vi "tlc_timer_main.vi"(7 "Command (Check Timer)":T1=enum."Check Timer", 8 "error in (no error)":errorcluster, 11 "Target Time (s)":dbl) -> (0 "error out":errorcluster, 3 "Elapsed":bool)   [LabVIEW 2009]
doc: "This VI is the Main VI for the Timer module. The Timer module is responsible for checking whether the Target Time has Elapsed.\n\nSee Block Diagram for more detailed information."
uses:
  tlc_timer_Command_enum.ctl
panel:
  # "Inputs"
  # "Outputs"
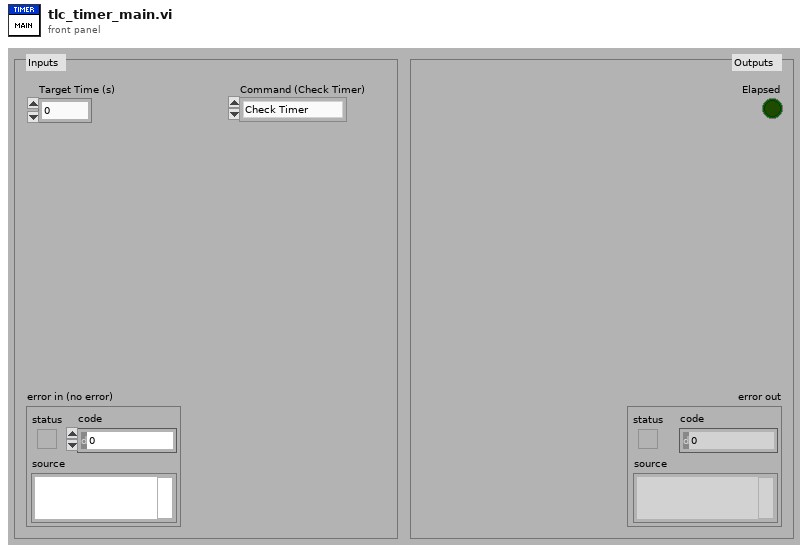
[diagram p1: front panel]
types:
  T1 = typedef "tlc_timer_Command_enum.ctl" = enum16{"Start Timer", "Check Timer"}
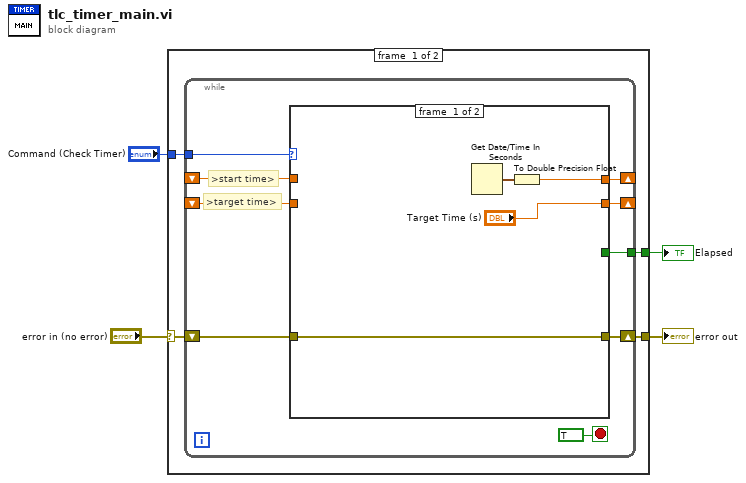
[diagram p0: block diagram]
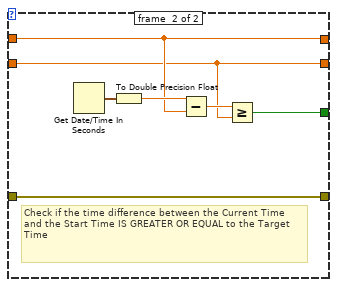
[diagram p2: hidden frame]
diagram:
  n1 = case shown="No Error" "error in (no error)" {
    selector: "error in (no error)" -> [w8 w29]
    tunnel: [w7 w29] -> w3
    tunnel: "Command (Check Timer)" -> [w6 _]
    tunnel: [w5 _] -> w1
    frame #0 {
      n2 = while {
        shift-right: [w17] -> w7
        shift-left: w8 -> [w16]
        tunnel: w6 -> [w15]
        shift-right: [w13] -> _
        shift-left: _ -> [w14]
        tunnel: [w12] -> w5
        shift-right: [w9] -> _
        shift-left: _ -> [w10]
        stop <- TRUE stop-if-true
        # ">target time>"
        # ">start time>"
        n3 = case shown="\"Check Timer\"" w15 {
          tunnel: [w21 w28] -> w17
          tunnel: w16 -> [w21 w28]
          tunnel: w14 -> [_ w23]
          tunnel: [w19 w23] -> w13
          tunnel: [_ w24] -> w12
          tunnel: w10 -> [_ w22]
          tunnel: ["Target Time (s)" w22] -> w9
          frame #0 {
            n4 = Get Date/Time In Seconds() -> (seconds since 1Jan1904=w20:timestamp)
            n5 = To Double Precision Float(number=w20) -> (double precision float=w19:dbl)
          }
          frame #1 {
            # "Check if the time difference between the Current Time and the Start Time IS GREATER OR EQUAL to the Target Time"
            n6 = Get Date/Time In Seconds() -> (seconds since 1Jan1904=w27:timestamp)
            n7 = To Double Precision Float(number=w27) -> (double precision float=w26:dbl)
            n8 = Subtract(x=w26, y=w23) -> (x-y=w25:dbl)
            n9 = Greater Or Equal?(x=w25, y=w22) -> (x >= y?=w24:bool)
          }
        }
      }
    }
    frame #1 {
    }
  }
  "error out" <- w3
  "Elapsed" <- w1
